vi "VRM.Ramp to Zero.vi"(6 "Axis":T1=enum."Z", 8 "error in (no error)":errorcluster, 11 "Instrument.VRM in":refnum<class "Instrument.OxfordVRM.lvclass">) -> (0 "error out":errorcluster, 2 "Response":string[](array[string]), 3 "Instrument.VRM out":refnum<class "Instrument.OxfordVRM.lvclass">)   [LabVIEW 2019]
uses:
  Instrument.OxfordVRM.lvclass
  <instrlib>/Mercury iXX/Public/Libraries/Magnet/Controls/PSU Actions.ctl
  <instrlib>/Mercury iXX/Public/Libraries/Magnet.lvlib
  Typedefs/VRM Magnet Axis--Enum.ctl
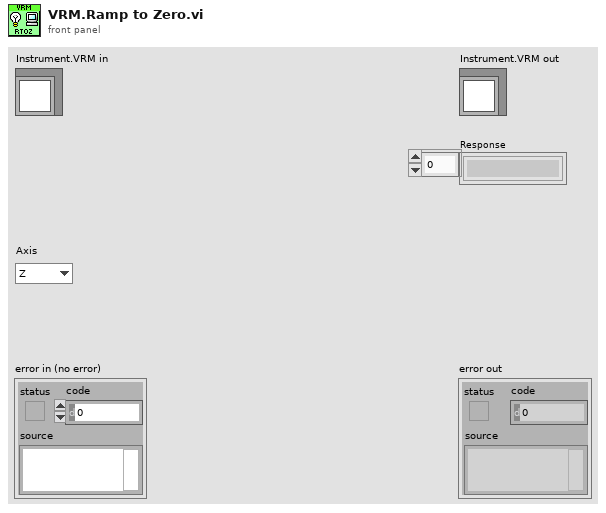
[diagram p1: front panel]
types:
  T1 = typedef "Instrument.OxfordVRM.lvclass/VRM Magnet Axis--Enum.ctl" = enum16{"X", "Y", "Z", "ALL"}
  T2 = typedef "Mercury iXX.lvlib/Magnet.lvlib/PSU Actions.ctl" = string
  T3 = typedef "Instrument.Cryostat.lvclass/Magnet Axis--Enum.ctl" = enum16{"X", "Y", "Z"}
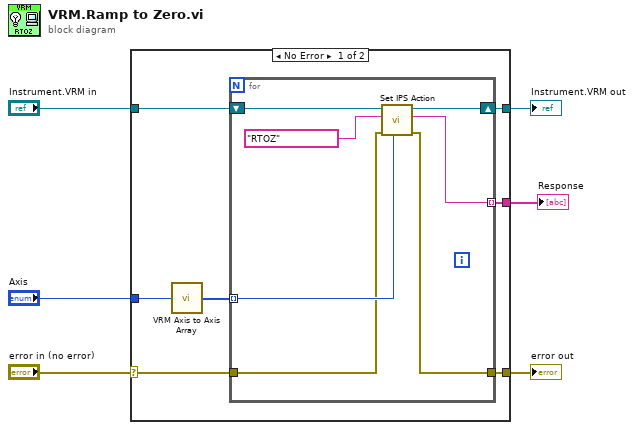
[diagram p0: block diagram]
diagram:
  n1 = case shown="No Error" "error in (no error)" {
    selector: "error in (no error)" -> [w12 w22]
    tunnel: [w10 w22] -> w5
    tunnel: [w11 w21] -> w3
    tunnel: "Instrument.VRM in" -> [w13 w21]
    tunnel: "Axis" -> [w8 _]
    tunnel: [w7 _] -> w1
    frame No Error {
      n2 = call "VRM Axis to Axis Array.vi"("Axis"=w8) -> ("Axis Array"=w9:T3[])
      n3 = for {
        shift-right: [w19] -> w11
        shift-left: w13 -> [w20]
        tunnel: w9 -> [w17] mode=indexing
        tunnel: w12 -> [w16]
        tunnel: [w15] -> w10
        tunnel: [w14] -> w7 mode=indexing
        n4 = call "Set IPS Action.vi"("Axis"=w17, "error in (no error)"=w16, "PSU Act Stat"=T2 "RTOZ", "Instrument.OxfordVRM in"=w20) -> ("error out"=w15:errorcluster, "Response"=w14:string, "Instrument.OxfordVRM out"=w19:refnum<class "Instrument.OxfordVRM.lvclass">)  [unwired: 5 in]
      }
    }
    frame Error {
    }
  }
  "error out" <- w5
  "Instrument.VRM out" <- w3
  "Response" <- w1
